vi "Launch CS++StartActor.vi"(6 "CS++Classes & Messages":T1(array[cluster]), 8 "Error In":errorcluster, 9 "CS++Factory":path, 10 "Start Actor":string="CS++StartActor", 11 "DB Connection String":string) -> (0 "Error Out":errorcluster, 2 "Enqueuer of start Actor":refnum<class "Message Enqueuer.lvclass">, 3 "Attributes found?":bool=TRUE)   [LabVIEW 2015, in "CS++StartActor.lvlib"]
doc: "Launch CS++StartActor.\n\nUse command line parameters in case of Run Time System.\nDB=\"DB Connection String\"; Default:\"ApplicationName.ini\"\nFactory=\"Path to desired Factory class\"; Default: \"emptyString\" use CS++Factory \nStartActor=\"Name of desired start actor\"; Default: \"CS++StartActor\""
uses:
  CS++StartActor.lvlib
  <vilib>/ActorFramework/Message Enqueuer/Message Enqueuer.lvclass
  <vilib>/ActorFramework/Message/Message.lvclass
  Libraries/Base/FGV Action.ctl
  Classes/CS++BaseClasses/Factory/CS++Factory.lvclass
  Classes/CS++BaseClasses/Factory/CS++Factory.lvclass/CS++Factory.ctl
  Libraries/Base/CS++Base.lvlib
  Classes/CS++ProcessVariables/CS++ProcessVariables.lvlib
  <vilib>/ActorFramework/Actor/Actor.lvclass
panel:
  in  "Type":T2={"DB Connection String"="", "Start Actor"="CS++StartActor", "CS++Factory"=path ""}
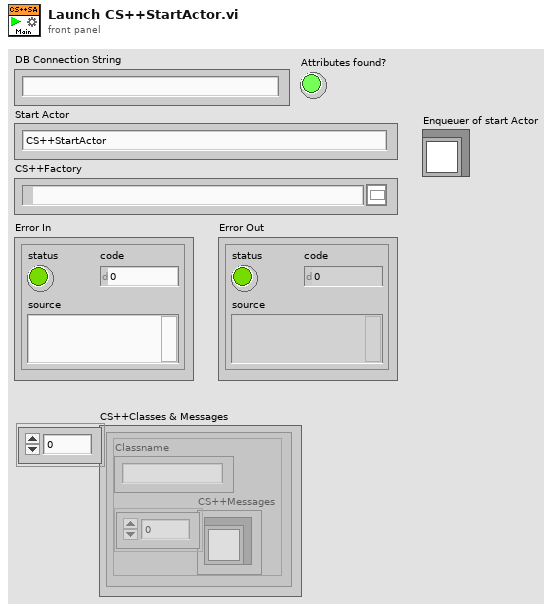
[diagram p1: front panel]
types:
  T1 = cluster{"Classname":string, "CS++Messages":refnum<class "Message.lvclass">[]}[]
  T2 = cluster{"DB Connection String":string, "Start Actor":string, "CS++Factory":path}
  T3 = typedef "CS++Base.lvlib/FGV Action.ctl" = enum16{"add", "replace", "read", "remove", "reset", "get attributes"}
  T4 = enum32{"invalid app kind", "Development System", "Run Time System", "Student Edition", "Embedded LabVIEW", "Evaluation", "Custom"}
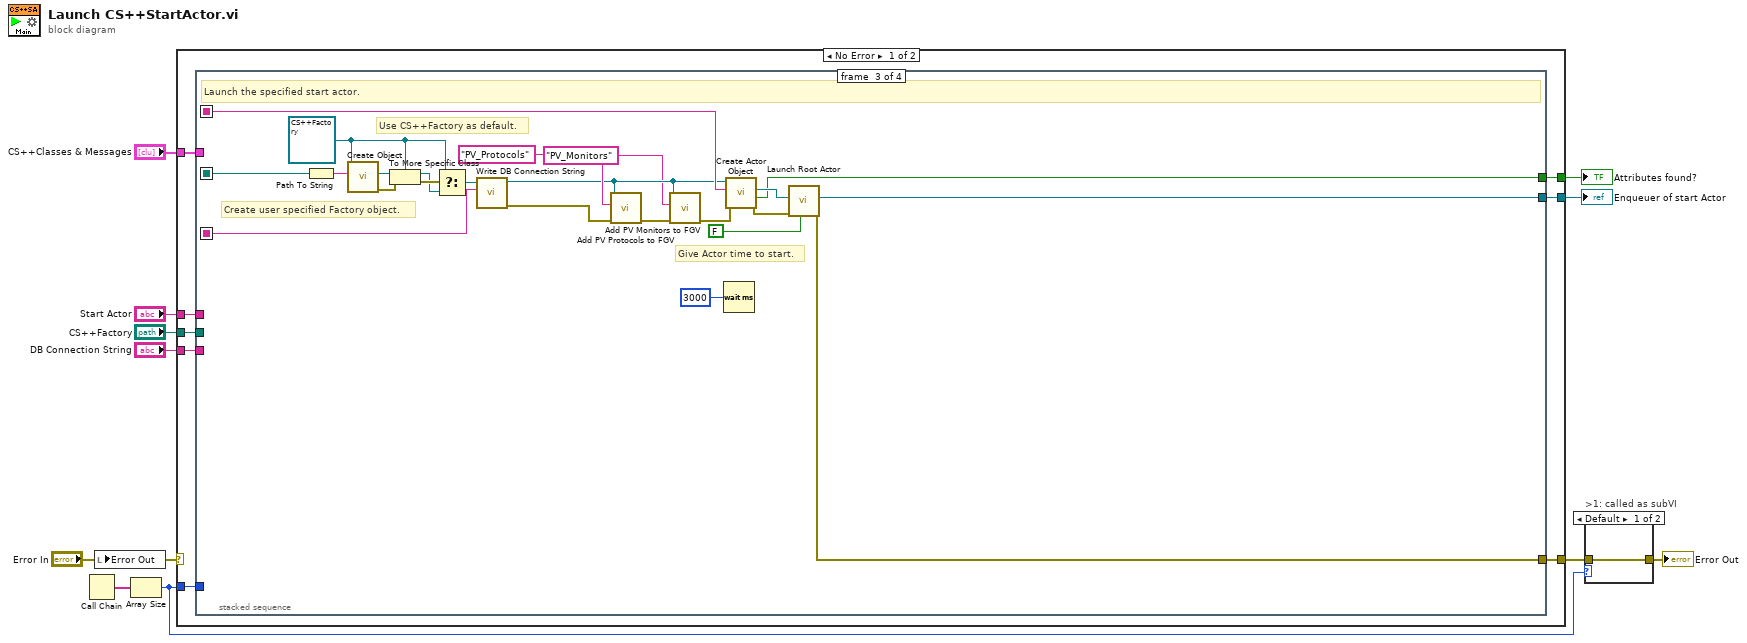
[diagram p0: block diagram]
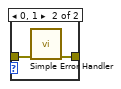
[diagram p2: hidden frame]
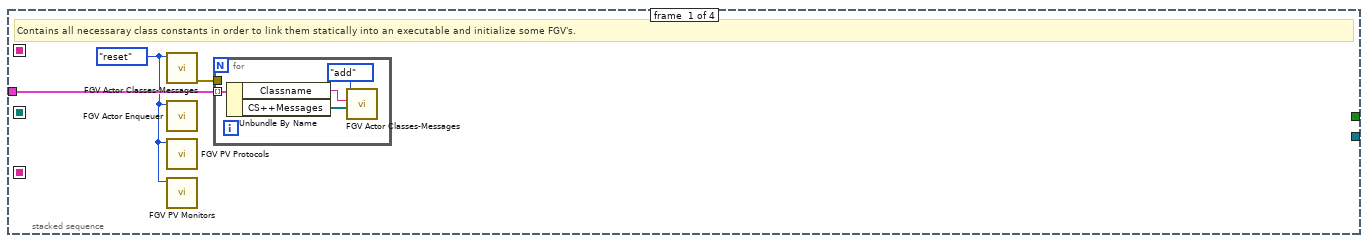
[diagram p3: hidden frame]
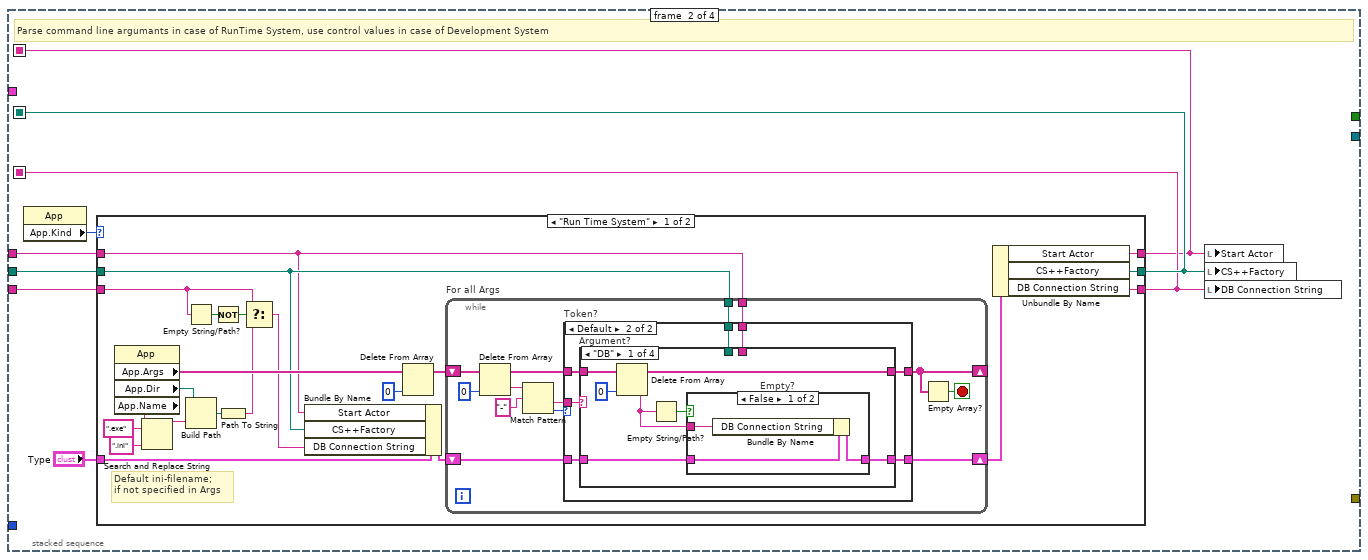
[diagram p4: hidden frame]
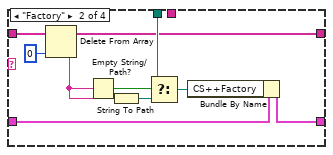
[diagram p7: hidden frame]
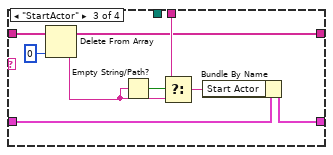
[diagram p8: hidden frame]
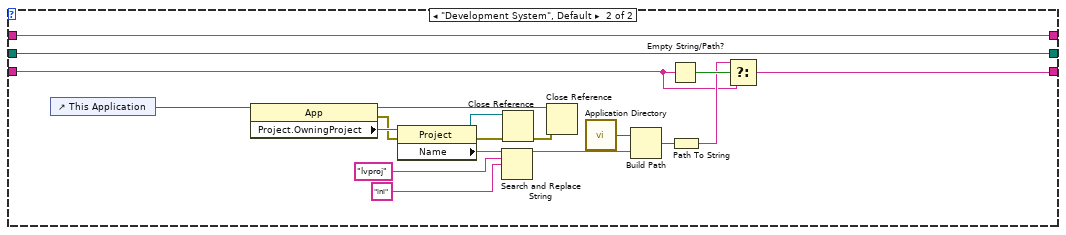
[diagram p10: hidden frame]
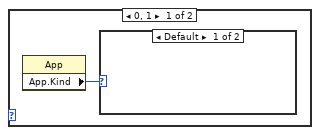
[diagram p12: hidden frame]
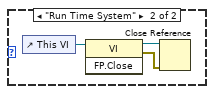
[diagram p13: hidden frame]
diagram:
  n1 = Call Chain() -> (call chain=w6:string[])
  n2 = local write "Error Out"("Error In") -> ()
  n3 = Array Size(array=w6) -> (size(s)=w5:i32)
  n4 = case shown="No Error" "Error In" {
    selector: "Error In" -> [_ w158]
    tunnel: [w16 w158] -> w11
    tunnel: "Start Actor" -> [w19 _]
    tunnel: "CS++Factory" -> [w18 _]
    tunnel: "DB Connection String" -> [w17 _]
    tunnel: w5 -> [w15 _]
    tunnel: [w14 _] -> w3
    tunnel: [w13 _] -> w2
    tunnel: "CS++Classes & Messages" -> [w12 _]
    frame No Error {
      n5 = stacked-sequence {
        seq-local: [_ w33 _ _] -> [_ _ w146 _]
        seq-local: [_ w34 _ _] -> [_ _ w144 _]
        seq-local: [_ w32 _ _] -> [_ _ w145 _]
        tunnel: w19 -> [_ w31 _ _]
        tunnel: w18 -> [_ w30 _ _]
        tunnel: w17 -> [_ w29 _ _]
        tunnel: [_ _ w137 _] -> w16
        tunnel: w15 -> [_ _ _ w153]
        tunnel: [_ _ w135 _] -> w14
        tunnel: [_ _ w130 _] -> w13
        tunnel: w12 -> [w21 _ _ _]
        frame #0 {
          w20 = FGV_Action."reset" ("Action (read)")
          # "Contains all necessaray class constants in order to link them statically into an executable and initialize some FGV's."
          n6 = call "FGV Actor Classes-Messages.vi"("Action (read)"=w20) -> ("Error Out"=w22:errorcluster)  [unwired: 6 in, 4 out]
          n7 = call "FGV Actor Enqueuer.vi"("Action (read)"=w20) -> ()  [unwired: 6 in, 5 out]
          n8 = call "FGV PV Protocols.vi"("Action (read)"=w20) -> ()  [unwired: 6 in, 5 out]
          n9 = call "FGV PV Monitors.vi"("Action (read)"=w20) -> ()  [unwired: 6 in, 5 out]
          n10 = for {
            tunnel: w21 -> [w25] mode=indexing
            tunnel: w22 -> [_]
            n11 = Unbundle By Name(w25) -> ("Classname"=w24:string, "CS++Messages"=w23:refnum<class "Message.lvclass">[])
            n12 = call "FGV Actor Classes-Messages.vi"("CS++Messages"=w23, "Class Name"=w24, "Action (read)"=FGV_Action."add") -> ()  [unwired: 4 in, 5 out]
          }
        }
        frame #1 {
          # "Parse command line argumants in case of RunTime System, use control values in case of Development System"
          n13 = property class="App"() -> ("App.Kind"=w28:T4)  [unwired: 2 in, 2 out]
          n14 = case shown="\"Run Time System\"" w28 {
            tunnel: [w48 w129] -> w32
            tunnel: w31 -> [w35 w129]
            tunnel: [w47 w128] -> w34
            tunnel: w30 -> [w36 w128]
            tunnel: [w46 w116] -> w33
            tunnel: w29 -> [w39 w117]
            tunnel: "Type" -> [w44 _]
            frame "Run Time System" {
              # "Default ini-filename;\nif not specified in Args"
              n15 = property class="App"() -> ("App.Args"=w42:string[], "App.Dir"=w52:path, "App.Name"=w51:string)  [unwired: 2 in, 2 out]
              n16 = Search and Replace String(input string=w51, search string=".exe", replace string=".ini" ("replace string (\"\")")) -> (result string=w55:string)  [unwired: 5 in, 3 out]
              n17 = Empty String/Path?(string/path=w39) -> (empty?=w41:bool)
              n18 = Build Path(base path=w52, name or relative path=w55) -> (appended path=w56:path)
              n19 = Not(x=w41) -> (.not. x?=w38:bool)
              n20 = Path To String(path=w56) -> (string=w37:string)
              n21 = Select(t=w39, s=w38, f=w37) -> (s? t:f=w40:string)
              n22 = Bundle By Name(cluster=w44, "Start Actor"=w35, "CS++Factory"=w36, "DB Connection String"=w40) -> (w43:T2)
              n23 = Delete From Array(array=w42, index=0) -> (array with subset deleted=w50:string[])  [unwired: 1 in, 1 out]
              n24 = while "For all Args" {
                shift-right: [w68] -> w49
                shift-left: w43 -> [w69]
                tunnel: w35 -> [w67]
                tunnel: w36 -> [w66]
                shift-right: [w61] -> _
                shift-left: w50 -> [w65]
                stop <- w62 stop-if-true
                n25 = Delete From Array(array=w65, index=0) -> (deleted portion=w60:string, array with subset deleted=w64:string[])  [unwired: 1 in]
                n26 = Match Pattern(string=w60, regular expression="-" ("search string/char (-)")) -> (after substring=w58:string, offset past match=w57:i32)  [unwired: 1 in, 2 out]
                n27 = case "Token?" shown="Default" w57 {
                  tunnel: w69 -> [w70 w78]
                  tunnel: [w70 w77] -> w68
                  tunnel: w67 -> [_ w76]
                  tunnel: w66 -> [_ w75]
                  tunnel: w58 -> [_ w74]
                  tunnel: w64 -> [w71 w73]
                  tunnel: [w71 w72] -> w61
                  frame -1 {
                  }
                  frame Default {
                    n28 = case "Argument?" shown="\"DB\"" w74 {
                      tunnel: w78 -> [w85 w99 w108 w110]
                      tunnel: [w84 w98 w107 w110] -> w77
                      tunnel: w76 -> [_ _ w104 _]
                      tunnel: w75 -> [_ w95 _ _]
                      tunnel: [w82 w91 w101 w109] -> w72
                      tunnel: w73 -> [w83 w92 w102 w109]
                      frame "DB" {
                        n29 = Delete From Array(array=w83, index=0) -> (deleted portion=w80:string, array with subset deleted=w82:string[])  [unwired: 1 in]
                        n30 = Empty String/Path?(string/path=w80) -> (empty?=w79:bool)
                        n31 = case "Empty?" shown="False" w79 {
                          tunnel: w85 -> [w88 w89]
                          tunnel: [w87 w89] -> w84
                          tunnel: w80 -> [w86 _]
                          frame False {
                            n32 = Bundle By Name(cluster=w88, "DB Connection String"=w86) -> (w87:T2)
                          }
                          frame True {
                          }
                        }
                      }
                      frame "Factory" {
                        n33 = Delete From Array(array=w92, index=0) -> (deleted portion=w90:string, array with subset deleted=w91:string[])  [unwired: 1 in]
                        n34 = Empty String/Path?(string/path=w90) -> (empty?=w97:bool)
                        n35 = String To Path(string=w90) -> (path=w94:path)
                        n36 = Select(t=w95, s=w97, f=w94) -> (s? t:f=w96:path)
                        n37 = Bundle By Name(cluster=w99, "CS++Factory"=w96) -> (w98:T2)
                      }
                      frame "StartActor" {
                        n38 = Delete From Array(array=w102, index=0) -> (deleted portion=w100:string, array with subset deleted=w101:string[])  [unwired: 1 in]
                        n39 = Empty String/Path?(string/path=w100) -> (empty?=w106:bool)
                        n40 = Select(t=w104, s=w106, f=w100) -> (s? t:f=w105:string)
                        n41 = Bundle By Name(cluster=w108, "Start Actor"=w105) -> (w107:T2)
                      }
                      frame Default {
                      }
                    }
                  }
                }
                n42 = Empty Array?(array=w61) -> (empty?=w62:bool)
              }
              n43 = Unbundle By Name(w49) -> ("Start Actor"=w48:string, "CS++Factory"=w47:path, "DB Connection String"=w46:string)
            }
            frame "Development System", Default {
              n44 = control-ref of="This Application"() -> (w123:refnum<vi>)
              n45 = property class="App"(reference=w123) -> (reference out=w112:refnum<vi>, error out=w113:errorcluster, "Project.OwningProject"=w122:refnum<vi>)  [unwired: 1 in]
              n46 = property class="Project"(reference=w122, error in=w113) -> (reference out=w115:refnum<vi>, error out=w114:errorcluster, "Name"=w121:string)
              n47 = Search and Replace String(input string=w121, search string="lvproj" ("search string/char (-)"), replace string="ini" ("string")) -> (result string=w118:string)  [unwired: 5 in, 3 out]
              n48 = Close Reference(reference=w115, error in (no error)=w114) -> (error out=w111:errorcluster)
              n49 = Close Reference(reference=w112, error in (no error)=w111) -> ()  [unwired: 1 out]
              n50 = call <vilib>:"Application Directory.vi"() -> ("Application Directory"=w126:path)
              n51 = Build Path(base path=w126, name or relative path=w118) -> (appended path=w125:path)
              n52 = Empty String/Path?(string/path=w117) -> (empty?=w127:bool)
              n53 = Path To String(path=w125) -> (string=w124:string)
              n54 = Select(t=w124, s=w127, f=w117) -> (s? t:f=w116:string)
            }
          }
          n55 = local write "Start Actor"(w32) -> ()
          n56 = local write "CS++Factory"(w34) -> ()
          n57 = local write "DB Connection String"(w33) -> ()
        }
        frame #2 {
          w140 = refnum<class "CS++Factory.lvclass"> refnum ("CS++BaseClasses.lvlib:CS++Factory.lvclass")
          # "Use CS++Factory as default."
          # "Create user specified Factory object."
          # "Give Actor time to start."
          # "Launch the specified start actor."
          n58 = Path To String(path=w144) -> (string=w143:string)
          n59 = call "Create Object.vi"("Object Name"=w143, "CS++Factory in"=w140) -> ("error out"=w141:errorcluster, "LabVIEW Object"=w142:refnum<class>)  [unwired: 6 in, 2 out]
          n60 = To More Specific Class(target class=w140, reference=w142, error in=w141) -> (specific class reference=w148:refnum<class "CS++Factory.lvclass">, error out=w149:errorcluster)
          n61 = Select(t=w140, s=w149, f=w148) -> (s? t:f=w147:refnum<class "CS++Factory.lvclass">)
          n62 = call "Write DB Connection String.vi"("DB Connection String"=w146, "CS++Factory in"=w147) -> ("error out"=w139:errorcluster, "CS++Factory out"=w134:refnum<class "CS++Factory.lvclass">)  [unwired: 8 in]
          n63 = call "Add PV Protocols to FGV.vi"("Error In"=w139, "PV Protocol Section"="PV_Protocols" ("string"), "CS++Factory"=w134) -> ("Error Out"=w133:errorcluster)  [unwired: 8 in]
          n64 = call "Add PV Monitors to FGV.vi"("Error In"=w133, "PV Monitor Section"="PV_Monitors", "CS++Factory"=w134) -> ("Error Out"=w132:errorcluster)  [unwired: 8 in]
          n65 = Wait (ms)(milliseconds to wait=u32 3000) -> ()  [unwired: 1 out]
          n66 = call "Create Actor Object.vi"("error in (no error)"=w132, "Object Name"=w145, "CS++Factory in"=w134) -> ("error out"=w150:errorcluster, "Attributes found?"=w135:bool, "CS++BaseActor"=w151:refnum<class "CS++BaseActor.lvclass">)  [unwired: 5 in, 1 out]
          n67 = call <vilib>:"Launch Root Actor.vi"("Open Actor Core front panel? (F)"=FALSE, "error in (no error)"=w150, "Actor"=w151) -> ("error out"=w137:errorcluster, "Actor's Enqueuer"=w130:refnum<class "Message Enqueuer.lvclass">)  [unwired: 7 in]
        }
        frame #3 {
          # "Close FP in case of Run Time System and not called as subVI."
          n68 = case ">1: called as subVI" shown="Default" w153 {
            frame 0, 1 {
              n69 = property class="App"() -> ("App.Kind"=w154:T4)  [unwired: 2 in, 2 out]
              n70 = case shown="Default" w154 {
                frame Default {
                }
                frame "Run Time System" {
                  n71 = control-ref of="This VI"() -> (w157:refnum<vi>)
                  n72 = invoke class="VI" method="FP.Close"(reference=w157) -> (reference out=w156:refnum<vi>, error out=w155:errorcluster)  [unwired: 2 in, 1 out]
                  n73 = Close Reference(reference=w156, error in (no error)=w155) -> ()  [unwired: 1 out]
                }
              }
            }
            frame Default {
            }
          }
        }
      }
    }
    frame Error {
    }
  }
  "Attributes found?" <- w3
  "Enqueuer of start Actor" <- w2
  n74 = case ">1: called as subVI" shown="Default" w5 {
    tunnel: w11 -> [w159 w161]
    tunnel: [w159 w160] -> w7
    frame Default {
    }
    frame 0, 1 {
      n75 = call <vilib>:"Simple Error Handler.vi"("error in (no error)"=w161) -> ("error out"=w160:errorcluster)  [unwired: 4 in, 4 out]
    }
  }
  "Error Out" <- w7
